vi "16fail-sub.vi"(3 "Number":u64) -> (1 "Single Digit Sum":u64)   [LabVIEW 2021]
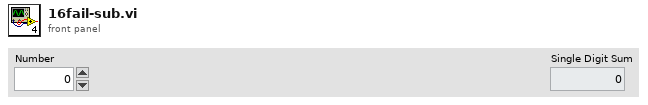
[diagram p1: front panel]
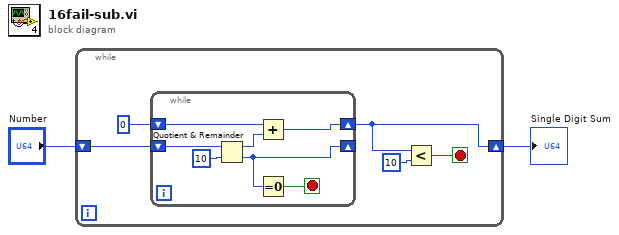
[diagram p0: block diagram]
diagram:
  n1 = while {
    shift-right: [w5] -> w1
    shift-left: "Number" -> [w7]
    stop <- w3 stop-if-true
    n2 = while {
      shift-right: [w11] -> w5
      shift-left: u64 0 -> [w9]
      shift-right: [w8] -> _
      shift-left: w7 -> [w13]
      stop <- w14 stop-if-true
      n3 = Quotient & Remainder(x=w13, y=u64 10) -> (x-y*floor(x/y)=w10:u64, floor(x/y)=w8:u64)
      n4 = Add(x=w9, y=w10) -> (x+y=w11:u64)
      n5 = Equal To 0?(x=w8) -> (x = 0?=w14:bool)
    }
    n6 = Less?(x=w5, y=u64 10) -> (x < y?=w3:bool)
  }
  "Single Digit Sum" <- w1
